vi "AVS_SetSyncMode.vi"(0 "a_hDevice":i32, 7 "a_Enable":u8) -> (4 "Output Value":i32)   [LabVIEW 2014, in "AvaSpec.lvlib" / "Avantes Spectrometer Functions.lvlib"]
uses:
  Avantes Spectrometer Functions.lvlib
  AS5216.dll
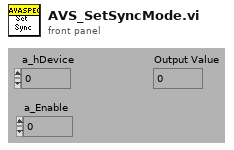
[diagram p1: front panel]
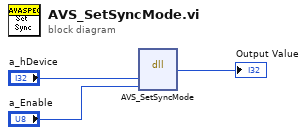
[diagram p0: block diagram]
diagram:
  n1 = dll-call lib="C:/Users/Daniel/Dropbox/CLTC/avantesSpectrometer/Libraries/AS-5216-DLL/polling_mc/AS5216.dll" fn="AVS_SetSyncMode"("a_hDevice"="a_hDevice", "a_Enable"="a_Enable") -> (→"Output Value":i32)  [unwired: 5 in, 2 out]
